vi "NULL State Queue.vi"() -> (0 "NULL State Queue":T1[](array[typedef]))   [LabVIEW 2013, in "State Machine Lib.lvlib"]
doc: "Returns an empty state queue."
uses:
  State Machine Lib.lvlib
  STATE cluster.ctl
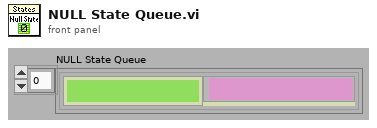
[diagram p1: front panel]
types:
  T1 = typedef "State Machine Lib.lvlib/STATE cluster.ctl" = cluster{"State":string, "Parameters":variant}
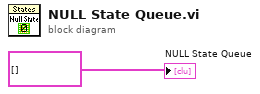
[diagram p0: block diagram]
diagram:
  "NULL State Queue" <- T1[] [] ("State que in")
